vi "SetZeroALL.vi"(10 "error in (no error)":errorcluster, 11 "reference":refnum<k24>) -> (2 "error out":errorcluster, 3 "new reference":refnum<k24>)   [LabVIEW 2017]
uses:
  C:/KMotion434/KMotion/Release/KMotion_dotNet.dll
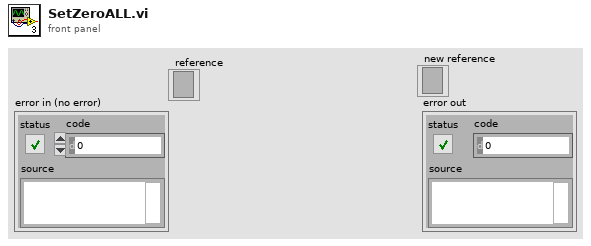
[diagram p1: front panel]
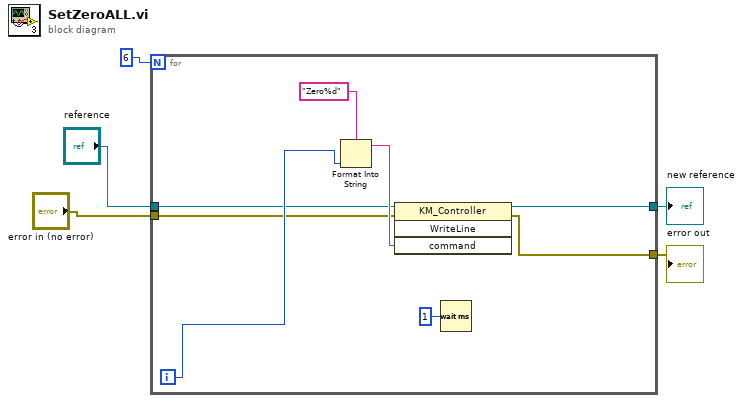
[diagram p0: block diagram]
diagram:
  n1 = for {
    N: 6 -> [_]
    tunnel: [w10] -> w4
    tunnel: [w9] -> w3
    tunnel: "error in (no error)" -> [w8]
    tunnel: "reference" -> [w7]
    i -> [w12]
    n2 = Format Into String(format string="Zero%d", w12) -> (resulting string=w13:string)  [unwired: 2 in, 1 out]
    n3 = invoke class="KM_Controller" method="WriteLine"(reference=w7, error in=w8, "command"=w13) -> (reference out=w10:refnum<k24>, error out=w9:errorcluster)  [unwired: 1 in, 2 out]
    n4 = Wait (ms)(milliseconds to wait=u32 1) -> ()  [unwired: 1 out]
  }
  "new reference" <- w4
  "error out" <- w3
